vi "Run Test.vi"(8 "error in (no error)":errorcluster, 11 "Test Template in":refnum<class "LCM Single-Up MTS Programming.lvclass">) -> (0 "error out":errorcluster, 1 "Fail Codes":string[](array[string]), 2 "Tests Passed":bool[](array[boolean]), 3 "Test Template out":refnum<class "LCM Single-Up MTS Programming.lvclass">)   [LabVIEW 2015, in "LCM Single-Up MTS Programming.lvclass"]
uses:
  LCM Single-Up MTS Programming.lvclass
  <vilib>/Cree, Inc/Cree Test Framework/Core Launcher/Core Manager Methods -- Enum.ctl
  Test Class/Test Class.lvclass/Test Class.ctl
  Test Class/Test Class.lvclass
  Classes/Application/Class/Application.lvclass
  <vilib>/Cree, Inc/Cree Test Framework/Core Launcher/Core Launcher.lvlib
  <vilib>/Cree, Inc/Cree Test Framework/Classes/Data/Data Repo/Class/Data Repo.lvclass
  LCM Single-Up Power Up/LCM Single-Up Power Up.lvclass
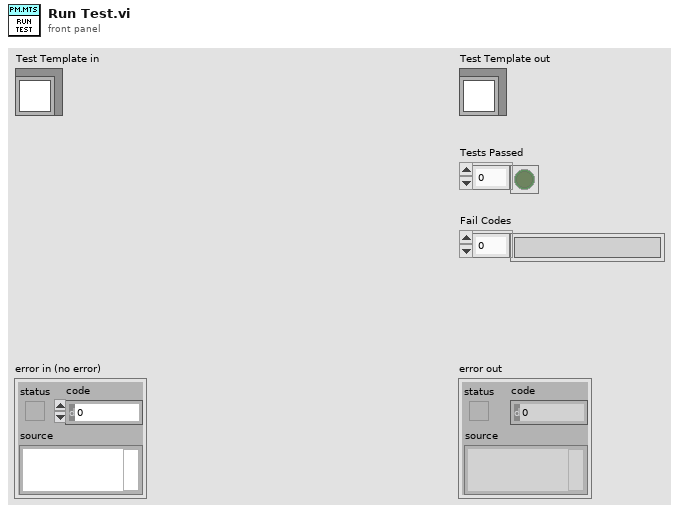
[diagram p1: front panel]
types:
  T1 = typedef "Core Launcher.lvlib/Core Manager Methods -- Enum.ctl" = enum16{"Spawn Objects", "Get Objects", "Destroy Objects"}
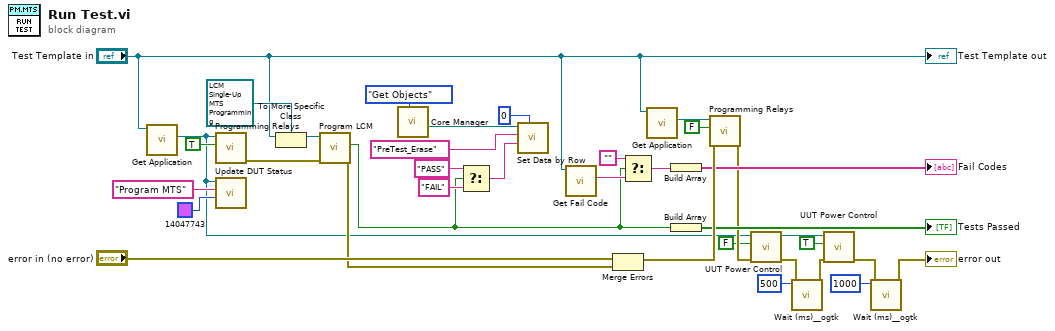
[diagram p0: block diagram]
diagram:
  n1 = call "Get Application.vi"("Test Class in"="Test Template in") -> ("Application.lvlib:Application.lvclass"=w4:refnum<class "Application.lvclass">)  [unwired: 9 in, 1 out]
  n2 = call "Programming Relays.vi"("Connect (False)"=TRUE, "Application in"=w4) -> ("error out"=w13:errorcluster)  [unwired: 9 in]
  n3 = call "Update DUT Status.vi"("BG Color"=u32 14047743, "Message ('')"="Program MTS", "Application in"=w4) -> ()  [unwired: 7 in, 2 out]
  n4 = To More Specific Class(target class=refnum<class "LCM Single-Up MTS Programming.lvclass"> refnum ("LCM Single-Up MTS Programming in"), reference="Test Template in") -> (specific class reference=w16:refnum<class "LCM Single-Up MTS Programming.lvclass">)  [unwired: 1 in, 1 out]
  n5 = call "Program LCM.vi"("error in (no error)"=w13, "LCM Single-Up MTS Programming in"=w16) -> ("error out"=w12:errorcluster, "Success"=w11:bool)  [unwired: 7 in, 1 out]
  n6 = call <vilib>:"Core Manager.vi"("Method"=Core_Manager_Methods_--_Enum."Get Objects") -> ("Data Repo"=w30:refnum<class "Data Repo.lvclass">)  [unwired: 7 in, 3 out]
  n7 = Select(t="PASS" ("Name"), s=w11, f="FAIL" ("Name")) -> (s? t:f=w31:string)
  n8 = call <vilib>:"Set Data by Row.vi"("Row"=0, "Value"=w31, "Header"="PreTest_Erase" ("Name"), "Acrobat Template in"=w30) -> ()  [unwired: 6 in, 2 out]
  n9 = call "Get Fail Code.vi"("Test Class in"="Test Template in") -> ("Fail Code"=w20:string)  [unwired: 9 in, 1 out]
  n10 = Merge Errors("error in (no error)", w12) -> (w35:errorcluster)
  n11 = Select(t="", s=w11, f=w20) -> (s? t:f=w22:string)
  n12 = call "Get Application.vi"("Test Class in"="Test Template in") -> ("Application.lvlib:Application.lvclass"=w18:refnum<class "Application.lvclass">)  [unwired: 9 in, 1 out]
  n13 = Build Array(w22) -> (→"Fail Codes":string[])
  n14 = Build Array(w11) -> (→"Tests Passed":bool[])
  n15 = call "Programming Relays.vi"("error in (no error)"=w35, "Connect (False)"=FALSE, "Application in"=w18) -> ("error out"=w9:errorcluster)  [unwired: 8 in]
  n16 = call "UUT Power Control.vi"("error in (no error)"=w9, "Connect (False)"=FALSE, "Application in"=w4) -> ("error out"=w8:errorcluster)  [unwired: 8 in]
  n17 = call <userlib>:"Wait (ms)__ogtk.vi"("error in (no error)"=w8, "milliseconds to wait"=u32 500) -> ("error out"=w5:errorcluster)  [unwired: 8 in, 1 out]
  n18 = call "UUT Power Control.vi"("error in (no error)"=w5, "Connect (False)"=TRUE, "Application in"=w4) -> ("error out"=w2:errorcluster)  [unwired: 8 in]
  n19 = call <userlib>:"Wait (ms)__ogtk.vi"("error in (no error)"=w2, "milliseconds to wait"=u32 1000) -> ("error out"=→"error out":errorcluster)  [unwired: 8 in, 1 out]
  "Test Template out" <- "Test Template in"
